vi "initOTDR.vi"(0 "matrix":i32, 2 "matrixSize":u32, 3 "Res BW Units":enum16{"PM", "GHz"}(ring)=enum."GHz") -> (1 "timeInc (ns)":dbl format="%.2f", 4 "t_max (ns)":dbl format="%.2f", 5 "Windowed JM Cluster":cluster{"X0":dbl, "dX":dbl, "Data":dbl[][]} {"Data" format="%.2f"; "dX" format="%.2f"; "X0" format="%.2f"}, 6 "Cursor X1":dbl=-6.3125e-08 caption="X1" format="%.4f", 7 "Cursor X2":dbl=-6.3125e-08 caption="X2" format="%.4f", 8 "Retain Settings":bool, 9 "Sigma (ns)":dbl format="%.3f", 10 "Res. BW":dbl=838.8608 caption="Window Res BW" format="%.2f")   [LabVIEW 2012]
uses:
  bin/OVA32.dll
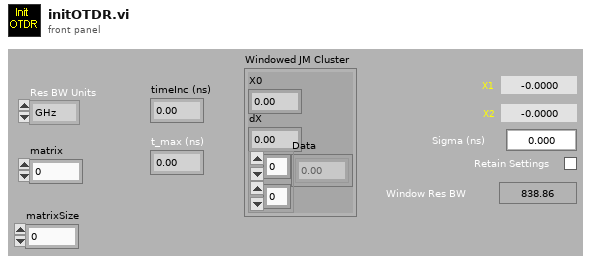
[diagram p1: front panel]
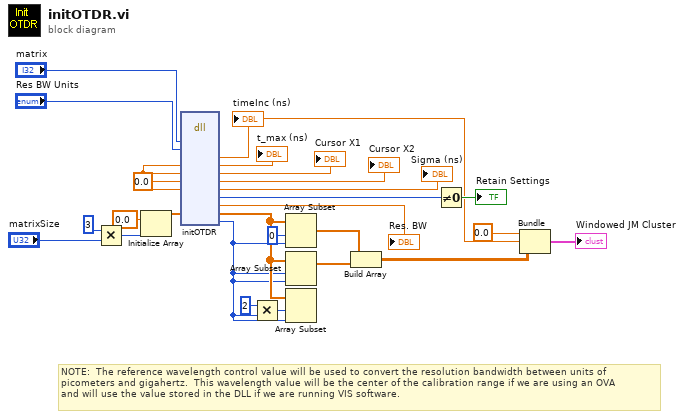
[diagram p0: block diagram]
diagram:
  w6 = 0.0
  # "NOTE:  The reference wavelength control value will be used to convert the resolution bandwidth between units of\npicometers and gigahertz.  This wavelength value will be the center of the calibration range if we are using an OVA\nand will use the value stored in the DLL if we are running VIS software."
  n1 = Multiply(x=3, y="matrixSize") -> (x*y=w17:u32)
  n2 = Initialize Array(0.0 ("Element Data"), w17) -> (w12:dbl[])
  n3 = dll-call lib="C:/_src/OVA5000_DSP_falcon/Software/LabVIEW/OVA/SDK/OVA_5000_SDK_v5.14.3/bin/OVA32.dll" fn="initOTDR"("matrix"="matrix", "units"="Res BW Units", "timeMax"=w6, "cursor1"=w6, "cursor2"=w6, "sigma"=w6, "window"=w12) -> ("timeInc"=w11:dbl, "timeMax"=→"t_max (ns)":dbl, "cursor1"=→"Cursor X1":dbl, "cursor2"=→"Cursor X2":dbl, "sigma"=→"Sigma (ns)":dbl, "retained"=w5:u8, "windowRSBW"=→"Res. BW":dbl, "window"=w3:dbl[], "windowSize"=w2:u32)  [unwired: 10 in, 2 out]
  "timeInc (ns)" <- w11
  n4 = Multiply(x=u32 2, y=w2) -> (x*y=w23:u32)
  n5 = Array Subset(array=w3, index=0 ("Array Index"), length=w2) -> (w26:dbl[])
  n6 = Array Subset(array=w3, index=w2, length=w2) -> (w25:dbl[])
  n7 = Array Subset(array=w3, index=w23, length=w2) -> ()  [unwired: 1 out]
  n8 = Build Array(w26, w25) -> (w24:dbl[][])
  n9 = Not Equal To 0?(x=w5) -> (x != 0?=→"Retain Settings":bool)
  n10 = Bundle(0.0, "timeInc"=w11, w24) -> (→"Windowed JM Cluster":cluster{dbl, "timeInc":dbl, dbl[][]})  [unwired: 1 in]
